vi "Inicializar.vi"(8 "error in (no error)":errorcluster, 11 "Simulada in":refnum<class "Simulada.lvclass">) -> (0 "error out":errorcluster, 3 "Simulada out":refnum<class "Simulada.lvclass">)   [LabVIEW 2020, in "Simulada.lvclass"]
uses:
  Simulada.lvclass
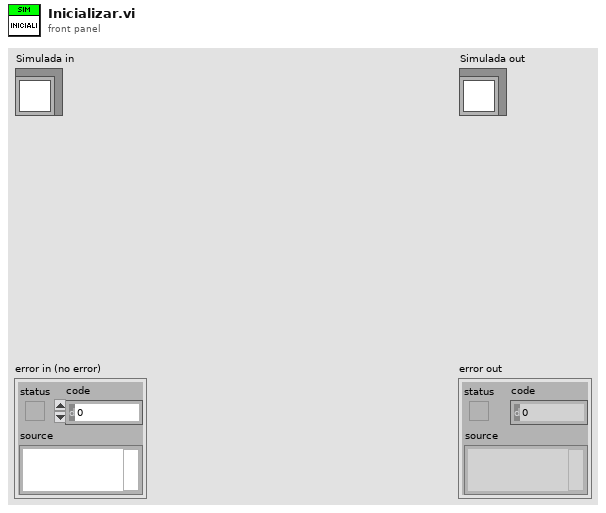
[diagram p1: front panel]
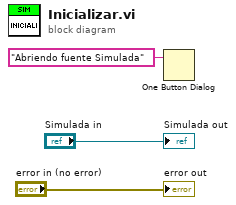
[diagram p0: block diagram]
diagram:
  n1 = One Button Dialog(message="Abriendo fuente Simulada") -> ()  [unwired: 1 in, 1 out]
  "error out" <- "error in (no error)"
  "Simulada out" <- "Simulada in"
